vi "Write Class Data to File.vi"(8 "error in":errorcluster, 10 "filter":u8, 11 "cCRDS Data in":refnum<class "cCRDS Data.lvclass">=refnum) -> (0 "error out":errorcluster, 2 "binFileOut":refnum<file>, 3 "cCRDS Data out":refnum<class "cCRDS Data.lvclass">)   [LabVIEW 2014, in "cCRDS Data.lvclass"]
uses:
  cCRDS Data.lvclass
  Reusable/CRDS/Data/Main/crd_data_enum.ctl
  cCRDS Data.lvclass/cCRDS Data.ctl
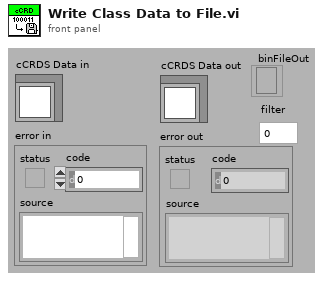
[diagram p1: front panel]
types:
  T1 = typedef "crd_data_enum.ctl" = enum8{"Time", "RHw", "TRH", "P", "Tmean", "RHsense", "TQ", "PQ", "Q", "Q0", "Qcal", "Qset", "extDilFac", "taucorr", "tau0corr", "stdevtau", "ext", "extCorr", "etau", "tau", "tau0", "Purge_Data", "NoData", "reserved", "Ttec", "Ang Exp", "Gamma", "filter", "fOverride", "notes", "max amp", "Tthermistor", "RhdilFac", "Psense", "TRHsense_bank", "RHsense_bank", "MFC_Data", "Thum", "ThumSP", "O3 Flow", "Pinlet Flow", "CLAP Flow", "O3 Add Valve", "O2 Valve", "O3 Cal"}
  T2 = enum16{"big-endian, network order", "native, host order", "little-endian"}
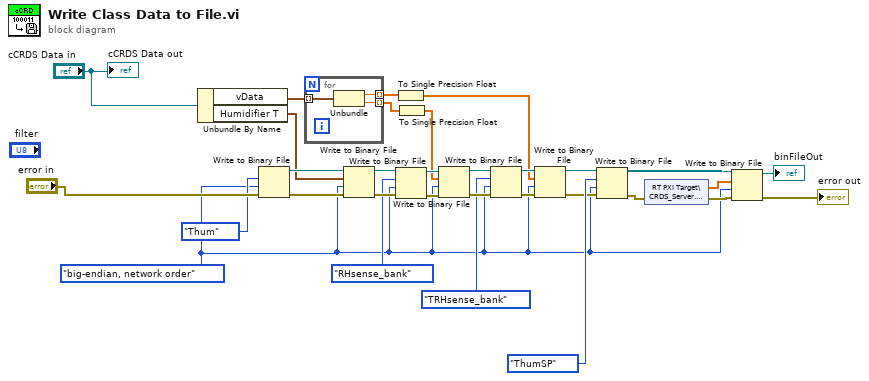
[diagram p0: block diagram]
diagram:
  w1 = T2."big-endian, network order" ("byte order (0:big-endian, network order)")
  n1 = Unbundle By Name("cCRDS Data in") -> ("vData"=w25:cluster{"TRH":dbl, "RH":dbl}[], "Humidifier T"=w26:cluster{"Hum 1":sgl, "Hum 2":sgl})
  n2 = Write to Binary File(data=crd_data_enum."Thum" ("CRD_Data_Enum"), error in="error in", 9:w1) -> (refnum out=w28:refnum<file>, error out=w27:errorcluster)  [unwired: 3 in, 1 out]
  n3 = for {
    tunnel: w25 -> [w34] mode=indexing
    tunnel: [w33] -> w21 mode=indexing
    tunnel: [w32] -> w20 mode=indexing
    n4 = Unbundle(w34) -> ("TRH"=w33:dbl, "RH"=w32:dbl)
  }
  n5 = Write to Binary File(file (use dialog)=w28, data=w26, error in=w27, 9:w1) -> (refnum out=w24:refnum<file>, error out=w23:errorcluster)  [unwired: 2 in, 1 out]
  n6 = To Single Precision Float(number=w21) -> (single precision float=w11:sgl[])
  n7 = Write to Binary File(file (use dialog)=w24, data=crd_data_enum."RHsense_bank" ("CRD_Data_Enum"), error in=w23, 9:w1) -> (refnum out=w19:refnum<file>, error out=w18:errorcluster)  [unwired: 2 in, 1 out]
  n8 = To Single Precision Float(number=w20) -> (single precision float=w17:sgl[])
  n9 = Write to Binary File(file (use dialog)=w19, data=w17, error in=w18, 9:w1) -> (refnum out=w16:refnum<file>, error out=w15:errorcluster)  [unwired: 2 in, 1 out]
  n10 = Write to Binary File(file (use dialog)=w16, data=crd_data_enum."TRHsense_bank" ("CRD_Data_Enum"), error in=w15, 9:w1) -> (refnum out=w14:refnum<file>, error out=w13:errorcluster)  [unwired: 2 in, 1 out]
  n11 = Write to Binary File(file (use dialog)=w14, data=w11, error in=w13, 9:w1) -> (refnum out=w9:refnum<file>, error out=w8:errorcluster)  [unwired: 2 in, 1 out]
  n12 = Write to Binary File(file (use dialog)=w9, data=crd_data_enum."ThumSP" ("CRD_Data_Enum"), error in=w8, 9:w1) -> (refnum out=w6:refnum<file>, error out=w3:errorcluster)  [unwired: 2 in, 1 out]
  n13 = shared-variable "RT PXI Target\\CRDS_Server.lvlib\\Tsp"(error in=w3) -> (w7:sgl[], error out=w2:errorcluster)
  n14 = Write to Binary File(file (use dialog)=w6, data=w7, error in=w2, 9:w1) -> (refnum out=→"binFileOut":refnum<file>, error out=→"error out":errorcluster)  [unwired: 2 in, 1 out]
  "cCRDS Data out" <- "cCRDS Data in"
